vi "Dequeue.vi"(6 "timeout (ms)":i32, 8 "error in (no error)":errorcluster) -> (0 "error out":errorcluster, 1 "Data":variant, 2 "Message":string)   [LabVIEW 2017, in "Messaging Library.lvlib"]
uses:
  Messaging Library.lvlib
  Controls/Q FGV States.ctl
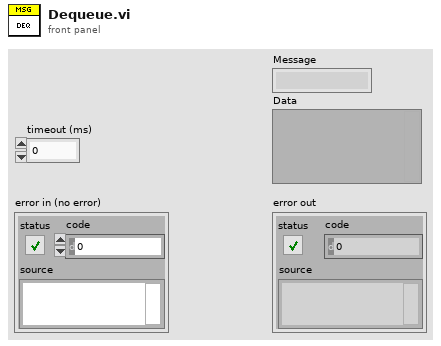
[diagram p1: front panel]
types:
  T1 = typedef "Messaging Library.lvlib/Q FGV States.ctl" = enum16{"Set", "Get"}
  T2 = typedef "Messaging Library.lvlib/Msg TypeDef.ctl" = cluster{"Message":string, "Data":variant}
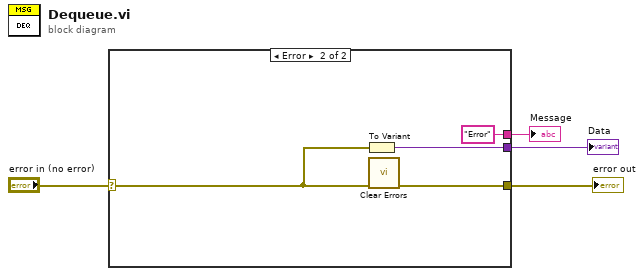
[diagram p0: block diagram]
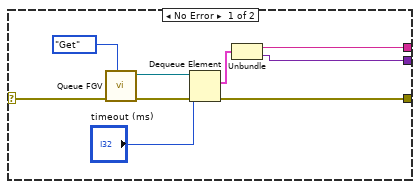
[diagram p2: hidden frame]
diagram:
  n1 = case shown="Error" "error in (no error)" {
    selector: "error in (no error)" -> [w8 w16]
    tunnel: [w13 w14] -> w3
    tunnel: [w7 w15] -> w2
    tunnel: [w6 "Error" ("Message")] -> w1
    frame No Error {
      n2 = call "Queue FGV.vi"("States"=Q_FGV_States."Get", "error in (no error)"=w8) -> ("error out"=w11:errorcluster, "Message Q Out"=w10:refnum<queue>)  [unwired: 8 in]
      n3 = Dequeue Element(queue=w10, timeout in ms (-1)="timeout (ms)", error in (no error)=w11) -> (element=w12:T2, error out=w13:errorcluster)  [unwired: 2 out]
      n4 = Unbundle(w12) -> ("Message"=w6:string, "Data"=w7:variant)
    }
    frame Error {
      n5 = To Variant(anything=w16) -> (Variant=w15:variant)
      n6 = call <vilib>:"Clear Errors.vi"("error in (no error)"=w16) -> ("error out"=w14:errorcluster)  [unwired: 5 in, 1 out]
    }
  }
  "error out" <- w3
  "Message" <- w1
  "Data" <- w2
